vi "Open Session.vi"(7 "Session Name ()":string, 8 "error in":errorcluster, 10 "Path":path) -> (0 "error out":errorcluster, 2 "created new?":bool, 3 "File DVR":T1)   [LabVIEW 2014, in "File Session.lvclass"]
doc: "Starts a new file session if one is not already present or retrieves a reference to one if one exists. If a session doees not exist AND the <b>Path</b> is not empty, then we will attempt to open a file."
uses:
  File Session.lvclass
  File Session DVR.ctl
  Create (Replace) File.vi
  <userlib>/_Session Fwk/Session - Root.lvclass
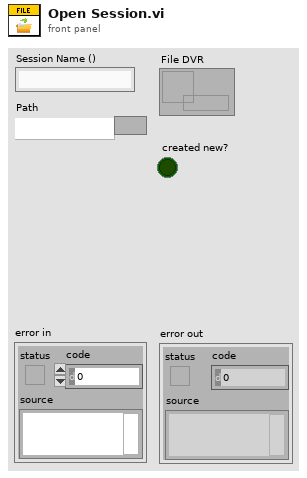
[diagram p1: front panel]
types:
  T1 = typedef "File Session.lvclass/File Session DVR.ctl" = refnum<data-value>
  T2 = typedef "Session - Root.lvclass/Session Handle.ctl" = refnum<data-value>
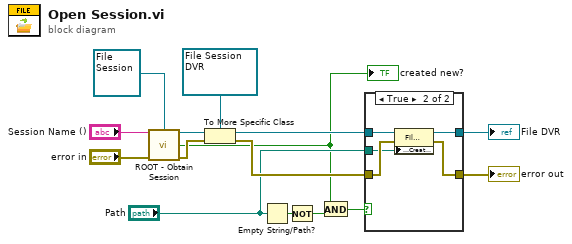
[diagram p0: block diagram]
diagram:
  n1 = call <userlib>:"ROOT - Obtain Session.vi"("Session Name ()"="Session Name ()", "OBJ - Session"=refnum<class "File Session.lvclass"> refnum ("File Session.lvclass"), "error in (no error)"="error in") -> ("Session Handle"=w15:T2, "created new?"=w2:bool, "error out"=w12:errorcluster)  [unwired: 10 in]
  "created new?" <- w2
  n2 = To More Specific Class(target class=T1 refnum ("File DVR"), reference=w15, error in=w12) -> (specific class reference=w9:T1, error out=w10:errorcluster)
  n3 = Empty String/Path?(string/path="Path") -> (empty?=w4:bool)
  n4 = Not(x=w4) -> (.not. x?=w3:bool)
  n5 = And(x=w2, y=w3) -> (x .and. y?=w1:bool)
  n6 = case shown="True" w1 {
    tunnel: "Path" -> [_ w18]
    tunnel: w10 -> [w16 w22]
    tunnel: w9 -> [w17 w21]
    tunnel: [w17 w20] -> w8
    tunnel: [w16 w19] -> w7
    frame False {
    }
    frame True {
      n7 = property class="File Session"(reference=w21, error in=w22, "Public:Create (Replace) File"=w18) -> (reference out=w20:T1, error out=w19:errorcluster)
    }
  }
  "error out" <- w7
  "File DVR" <- w8
